vi "TagContainer-Delete.vi"(8 "error in (no error)":errorcluster, 10 "name":string, 11 "TagContainer":T1) -> (0 "error out":errorcluster, 1 "found":bool, 3 "TagContainer(dup)":T1, 5 "Raw name":string)   [LabVIEW 2017, in "TagContainer.lvlib"]
uses:
  TagContainer.lvlib
  Typedef/TagContainer.ctl
panel:
  # "Connector Pane"
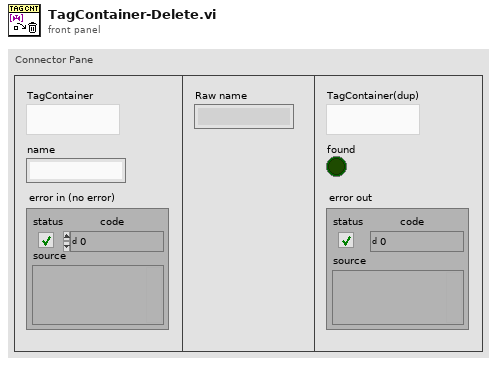
[diagram p1: front panel]
types:
  T1 = typedef "TagContainer.lvlib/TagContainer.ctl" = refnum<k1>
  T2 = typedef "TagContainer.lvlib/tagcontainer-data.ctl" = cluster{"tag-map":variant, "timestamp-map":variant, "namecacher-map":variant, "DataTypeCacher-map":variant, "Tag Adding Lock?":bool, "Global Change Timestamp":timestamp}
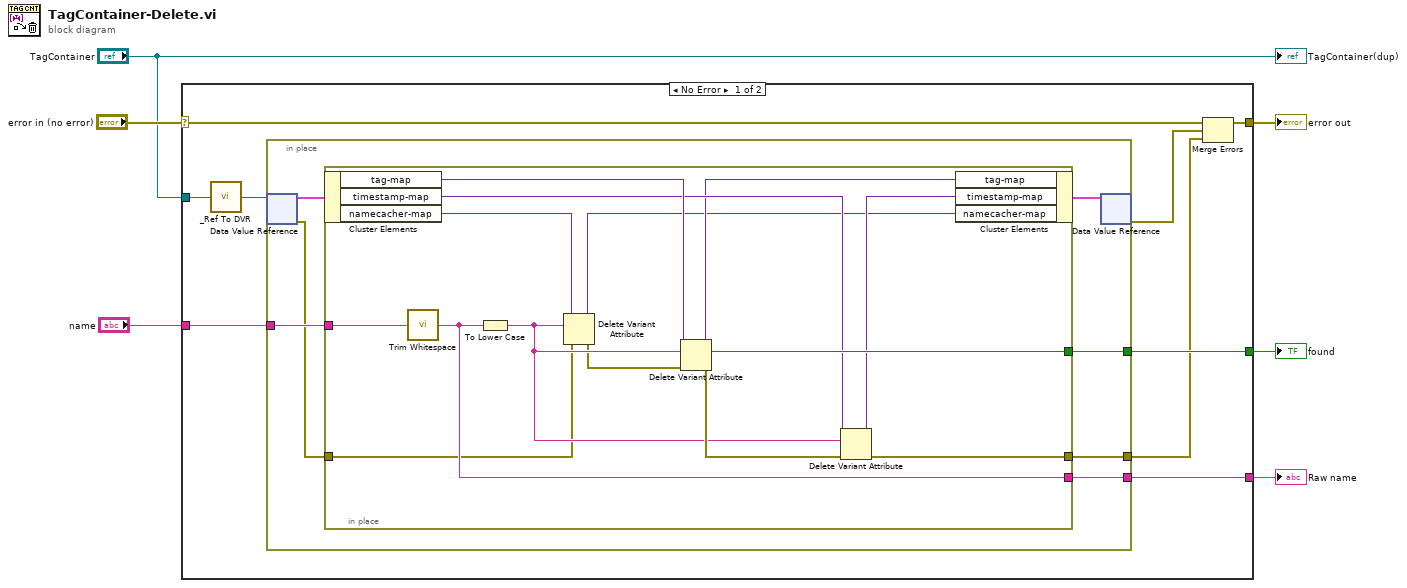
[diagram p0: block diagram]
diagram:
  n1 = case shown="No Error" "error in (no error)" {
    selector: "error in (no error)" -> [w14 w37]
    tunnel: [w15 w37] -> w5
    tunnel: "name" -> [w8 _]
    tunnel: "TagContainer" -> [w12 _]
    tunnel: [w11 _] -> w4
    tunnel: [w7 _] -> w1
    frame No Error {
      n2 = call "_Ref To DVR.vi"("TagContainer"=w12) -> ("DVR"=w10:refnum<data-value>)
      n3 = in-place "In Place Element Structure" {
        in-place-border: [w22] -> w11
        in-place-border: [w21] -> w9
        in-place-border: w8 -> [w20]
        in-place-border: [w19] -> w7
        n4 = in-place-dvr #1(w10) -> (w18:T2, w16:errorcluster)
        n5 = in-place {
          in-place-border: [w36] -> w22
          in-place-border: [w35] -> w21
          in-place-border: w20 -> [w34]
          in-place-border: [w26] -> w19
          in-place-border: w16 -> [w24]
          n6 = in-place-cluster #2(w18) -> ("tag-map"=w33:variant, "timestamp-map"=w32:variant, "namecacher-map"=w31:variant)
          n7 = call <vilib>:"Trim Whitespace.vi"("string"=w34) -> ("trimmed string"=w26:string)  [unwired: 1 in]
          n8 = To Lower Case(string=w26) -> (all lower case string=w25:string)
          n9 = Delete Variant Attribute(4:w24, 6:w25, 7:w31) -> (0:w23:errorcluster, 3:w28:variant)  [unwired: 1 out]
          n10 = Delete Variant Attribute(4:w23, 6:w25, 7:w33) -> (0:w27:errorcluster, 2:w36:bool, 3:w30:variant)
          n11 = Delete Variant Attribute(4:w27, 6:w25, 7:w32) -> (0:w35:errorcluster, 3:w29:variant)  [unwired: 1 out]
          n12 = in-place-cluster #2("tag-map"=w30, "timestamp-map"=w29, "namecacher-map"=w28) -> (w17:T2)
        }
        n13 = in-place-dvr #1(w17) -> (w13:errorcluster)  [unwired: 1 out]
      }
      n14 = Merge Errors(w14, w13, w9) -> (w15:errorcluster)
    }
    frame Error {
    }
  }
  "error out" <- w5
  "found" <- w4
  "Raw name" <- w1
  "TagContainer(dup)" <- "TagContainer"
